vi "TCP Daemon.vi"(8 "UUID":string, 9 "Data Model":refnum<class "Device Data Model.lvclass">, 11 "TCP slave in":refnum<class "TCP Server.lvclass">) -> ()   [LabVIEW 2021, in "WebSockets.lvlib" / "TCP Server.lvclass"]
doc: "This daemon waits for new connections and launches connection handlers as needed. It also obtains a local reference to the quit notification, and waits for that to occur."
uses:
  TCP Server.lvclass
  D:/my_projects/projects/Algorithms/Labview/21/WebSockets/Source/WebSockets/WebSocket Server/WebSocket Server.lvclass
  D:/my_projects/projects/Algorithms/Labview/21/WebSockets/Source/WebSockets/WebSocket/WebSocket.lvclass
  Modbus_v121c/Data Model/Device Data Model.lvclass
  Sockets/VISA TCP Socket/VISA TCP.lvclass
  daemon status.ctl
  Listener State.ctl
  WebSocket Server.lvclass/WebSocket Server.ctl
  TCP Server.lvclass/TCP Server.ctl
  WebSocket/WebSocket.lvclass/WebSocket.ctl
  Sockets/VISA TCP Socket/VISA TCP.lvclass/VISA TCP.ctl
  Read Port.vi
  Sockets/VISA TCP Socket/Read port.vi
  Remove Unused Connections.vi
  WebSocket Server.lvclass
  WebSocket/WebSocket.lvclass
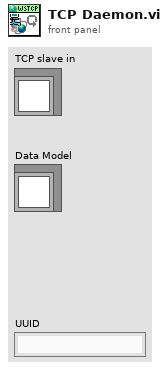
[diagram p1: front panel]
types:
  T1 = typedef "WebSockets.lvlib/WebSocket Server.lvclass/daemon status.ctl" = enum16{"Not Started", "Running", "Error", "Stopped"}
  T2 = typedef "WebSockets.lvlib/TCP Server.lvclass/Listener State.ctl" = enum16{"Check Notifier", "Check for Available Connection Slot", "Wait on Connection", "Quit"}
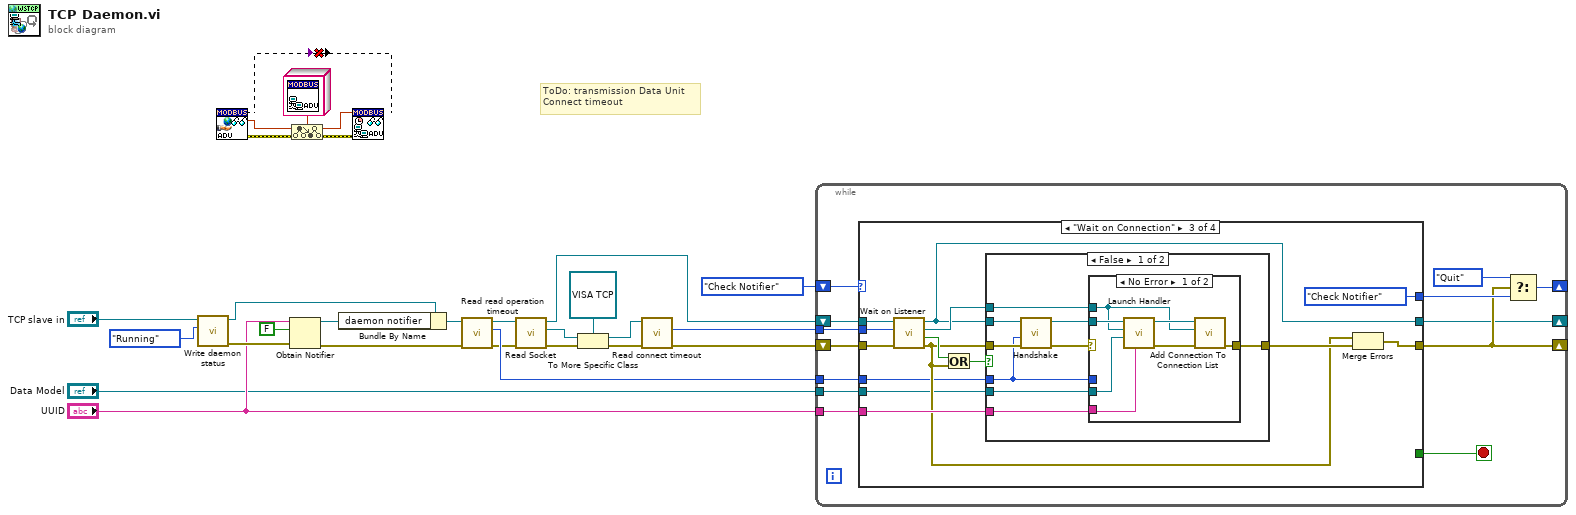
[diagram p0: block diagram]
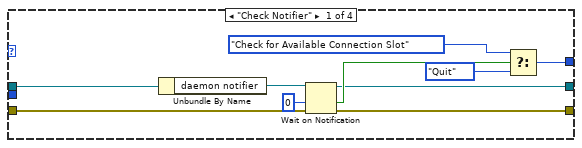
[diagram p2: hidden frame]
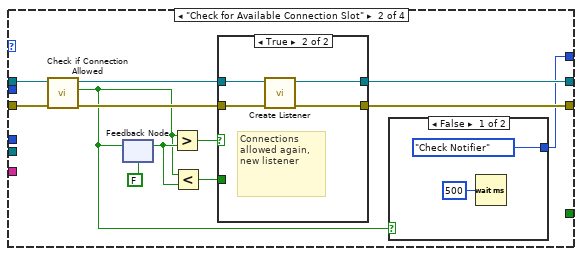
[diagram p3: hidden frame]
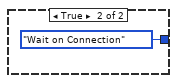
[diagram p4: hidden frame]
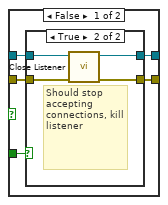
[diagram p5: hidden frame]
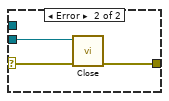
[diagram p7: hidden frame]
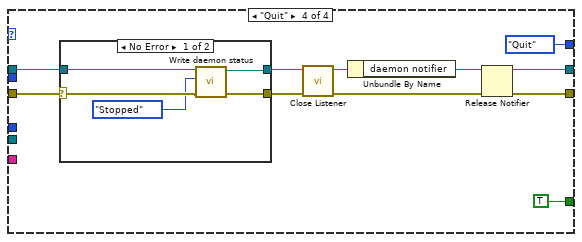
[diagram p9: hidden frame]
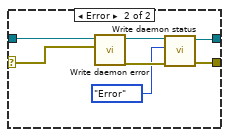
[diagram p10: hidden frame]
diagram:
  # "ToDo: transmission Data Unit \nConnect timeout"
  n1 = call "Write daemon status.vi"("daemon status"=daemon_status."Running", "WebSocket Server in"="TCP slave in") -> ("error out"=w19:errorcluster, "WebSocket Server out"=w16:refnum<class "TCP Server.lvclass">)  [unwired: 8 in]
  n2 = Obtain Notifier(name (unnamed)="UUID", notification data type=FALSE, error in (no error)=w19) -> (notifier out=w20:refnum<notifier>, error out=w7:errorcluster)  [unwired: 1 in, 1 out]
  n3 = Bundle By Name(cluster=w16, "daemon notifier"=w20) -> (w8:refnum<class "TCP Server.lvclass">)
  n4 = call "Read read operation timeout.vi"("error in (no error)"=w7, "Socket in"=w8) -> ("error out"=w5:errorcluster, "read operation timeout"=w9:i32, "Socket out"=w6:refnum<class "TCP Server.lvclass">)  [unwired: 7 in]
  n5 = call "Read Socket.vi"("error in (no error)"=w5, "WebSocket in"=w6) -> ("error out"=w4:errorcluster, "Socket"=w3:refnum<class "Socket.lvclass">, "WebSocket out"=w2:refnum<class "TCP Server.lvclass">)  [unwired: 7 in]
  n6 = To More Specific Class(target class=refnum<class "VISA TCP.lvclass"> refnum ("Sockets:VISA TCP"), reference=w3, error in=w4) -> (specific class reference=w12:refnum<class "VISA TCP.lvclass">, error out=w14:errorcluster)
  n7 = call "Read connect timeout.vi"("error in (no error)"=w14, "VISA TCP in"=w12) -> ("error out"=w10:errorcluster, "connect timeout"=w11:i32)  [unwired: 7 in, 1 out]
  n8 = while {
    shift-right: [w33] -> _
    shift-left: Listener_State."Check Notifier" -> [w35]
    tunnel: "UUID" -> [w30]
    shift-right: [w29] -> _
    shift-left: w10 -> [w28]
    shift-right: [w26] -> _
    shift-left: w2 -> [w34]
    tunnel: w11 -> [w25]
    tunnel: w9 -> [w24]
    tunnel: "Data Model" -> [w23]
    stop <- w27 stop-if-true
    n9 = case shown="\"Wait on Connection\"" w35 {
      tunnel: w34 -> [w36 w55 w87 w115]
      tunnel: [w43 w49 w81 w113] -> w29
      tunnel: [w38 w45 Listener_State."Check Notifier" Listener_State."Quit"] -> w31
      tunnel: w30 -> [_ _ w83 _]
      tunnel: w28 -> [w37 w56 w82 w116]
      tunnel: [_ _ _ TRUE] -> w27
      tunnel: [w36 w50 w76 w108] -> w26
      tunnel: w25 -> [_ _ w79 _]
      tunnel: w24 -> [_ _ w77 _]
      tunnel: w23 -> [_ _ w75 _]
      frame "Check Notifier" {
        n10 = Unbundle By Name(w36) -> ("daemon notifier"=w44:refnum<notifier>)
        n11 = Wait on Notification(notifier=w44, timeout in ms (-1)=0, error in (no error)=w37) -> (timed out?=w42:bool, error out=w43:errorcluster)  [unwired: 1 in, 2 out]
        n12 = Select(t=Listener_State."Check for Available Connection Slot", s=w42, f=Listener_State."Quit") -> (s? t:f=w38:T2)
      }
      frame "Check for Available Connection Slot" {
        n13 = call "Check if Connection Allowed.vi"("error in (no error)"=w56, "TCP Slave in"=w55) -> ("error out"=w52:errorcluster, "Connection Allowed"=w46:bool, "TCP Slave out"=w51:refnum<class "TCP Server.lvclass">)  [unwired: 7 in]
        n14 = feedback-in #1(w46) -> ()
        n15 = feedback #1(FALSE) -> (w48:bool)
        n16 = Greater?(x=w46, y=w48) -> (0:w53:bool)
        n17 = Less?(x=w46, y=w48) -> (x < y?=w47:bool)
        n18 = case shown="True" w53 {
          tunnel: w52 -> [w62 w73]
          tunnel: w51 -> [w63 w74]
          tunnel: [w60 w72] -> w50
          tunnel: [w61 w71] -> w49
          tunnel: w47 -> [w64 _]
          frame False {
            n19 = case shown="True" w64 {
              tunnel: w63 -> [w66 w70]
              tunnel: w62 -> [w65 w69]
              tunnel: [w65 w68] -> w61
              tunnel: [w66 w67] -> w60
              frame False {
              }
              frame True {
                # "Should stop accepting connections, kill listener"
                n20 = call "Close Listener.vi"("error in"=w69, "TCP slave in"=w70) -> ("error out"=w68:errorcluster, "TCP slave out"=w67:refnum<class "TCP Server.lvclass">)  [unwired: 8 in]
              }
            }
          }
          frame True {
            # "Connections allowed again, new listener"
            n21 = call "Create Listener.vi"("error in"=w73, "TCP slave in"=w74) -> ("error out"=w71:errorcluster, "TCP slave out"=w72:refnum<class "TCP Server.lvclass">)  [unwired: 8 in]
          }
        }
        n22 = case shown="False" w46 {
          tunnel: [Listener_State."Check Notifier" Listener_State."Wait on Connection"] -> w45
          frame False {
            n23 = Wait (ms)(milliseconds to wait=u32 500) -> ()  [unwired: 1 out]
          }
          frame True {
          }
        }
      }
      frame "Wait on Connection" {
        n24 = call-dynamic "Wait on Listener.vi"("error in"=w82, "timeout ms (wait forever: -1)"=w79, "TCP slave in"=w87) -> ("error out"=w78:errorcluster, "Timed Out"=w86:bool, "connection reference"=w84:refnum<data-value>, "TCP slave out"=w76:refnum<class "TCP Server.lvclass">)  [unwired: 5 in]
        n25 = Or(x=w86, y=w78) -> (x .or. y?=w85:bool)
        n26 = case shown="False" w85 {
          tunnel: w84 -> [w95 _]
          tunnel: w76 -> [w94 _]
          tunnel: w83 -> [w97 _]
          tunnel: [w96 _] -> w80
          tunnel: w78 -> [w92 _]
          tunnel: w77 -> [w90 _]
          tunnel: w75 -> [w89 _]
          frame False {
            n27 = call-dynamic "Handshake.vi"("error in (no error)"=w92, "timeout ms (5000)"=w90, "WebSocket Connection in"=w94) -> ("error out"=w91:errorcluster, "WebSocket Connection out"=w93:refnum<class "TCP Server.lvclass">)  [unwired: 7 in]
            n28 = case shown="No Error" w91 {
              selector: w91 -> [_ w105]
              tunnel: w97 -> [w103 _]
              tunnel: [w102 w104] -> w96
              tunnel: w93 -> [w100 w106]
              tunnel: w95 -> [w99 _]
              tunnel: w90 -> [_ _]
              tunnel: w89 -> [w98 _]
              frame No Error {
                n29 = call "Launch Handler.vi"("UUID"=w103, "Data Model"=w98, "connection reference"=w99, "TCP slave"=w100) -> ("error out"=w101:errorcluster)  [unwired: 7 in]
                n30 = call "Add Connection To Connection List.vi"("error in"=w101, "data value reference"=w99, "TCP Slave in"=w100) -> ("error out"=w102:errorcluster)  [unwired: 8 in]
              }
              frame Error {
                n31 = call-dynamic "Close.vi"("error in (no error)"=w105, "WebSocket in"=w106) -> ("error out"=w104:errorcluster)  [unwired: 8 in, 1 out]
              }
            }
          }
          frame True {
          }
        }
        n32 = Merge Errors(w78, w80) -> (w81:errorcluster)
      }
      frame "Quit" {
        n33 = case shown="No Error" w116 {
          selector: w116 -> [w118 w123]
          tunnel: [w119 w125] -> w114
          tunnel: w115 -> [w121 w128]
          tunnel: [w120 w126] -> w107
          frame No Error {
            n34 = call "Write daemon status.vi"("error in (no error)"=w118, "daemon status"=daemon_status."Stopped", "WebSocket Server in"=w121) -> ("error out"=w119:errorcluster, "WebSocket Server out"=w120:refnum<class "TCP Server.lvclass">)  [unwired: 7 in]
          }
          frame Error {
            n35 = call "Write daemon error.vi"("daemon error"=w123, "Network Slave in"=w128) -> ("error out"=w124:errorcluster, "Network Slave out"=w127:refnum<class "TCP Server.lvclass">)  [unwired: 8 in]
            n36 = call "Write daemon status.vi"("error in (no error)"=w124, "daemon status"=daemon_status."Error", "WebSocket Server in"=w127) -> ("error out"=w125:errorcluster, "WebSocket Server out"=w126:refnum<class "TCP Server.lvclass">)  [unwired: 7 in]
          }
        }
        n37 = call "Close Listener.vi"("error in"=w114, "TCP slave in"=w107) -> ("error out"=w109:errorcluster, "TCP slave out"=w108:refnum<class "TCP Server.lvclass">)  [unwired: 8 in]
        n38 = Unbundle By Name(w108) -> ("daemon notifier"=w110:refnum<notifier>)
        n39 = Release Notifier(notifier=w110, error in (no error)=w109) -> (error out=w113:errorcluster)  [unwired: 1 in, 2 out]
      }
    }
    n40 = Select(t=Listener_State."Quit", s=w29, f=w31) -> (s? t:f=w33:T2)
  }
